vi "IPI_TotalCollect.vi"(11 "Outputs":string[](array[string])) -> (3 "数字":T1)   [LabVIEW 2015]
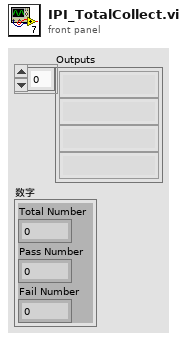
[diagram p1: front panel]
types:
  T1 = cluster{"Total Number":i32, "Pass Number":i32, "Fail Number":i32}
  T2 = cluster{"Total Number":string, "Pass Number":string, "Fail Number":string}
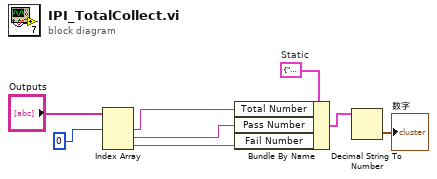
[diagram p0: block diagram]
diagram:
  w2 = T2 {"Total Number"="", "Pass Number"="", "Fail Number"=""}  # Static
  n1 = Index Array(array="Outputs", index #1=0 ("索引")) -> (element #1=w8:string, element #2=w7:string, element #3=w6:string)  [unwired: 2 in]
  n2 = Bundle By Name(cluster=w2, "Total Number"=w8, "Pass Number"=w7, "Fail Number"=w6) -> (w5:T2)
  n3 = Decimal String To Number(string=w5) -> (number=→"数字":T1)  [unwired: 2 in, 1 out]
